vi "Percent to Torque Request.vi"(9 "Enabled":bool, 11 "Throttle %":dbl) -> (2 "MTorqueRequest":sgl)   [LabVIEW 2014]
uses:
  Global Data.vi
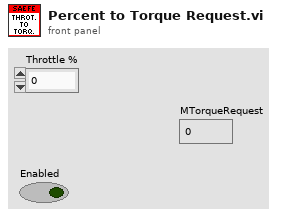
[diagram p1: front panel]
types:
  T1 = typedef "DashDriverInputs.ctl" = cluster{"ButtonsBitArray":u8, "NRedRotary":u8, "NYellowRotary":u8, "NBlackRotary":u8}
  T2 = typedef "MC Position.ctl" = cluster{"aMotor":dbl, "nMotor":dbl, "fMCOutput":dbl, "aDeltaResolverFilt":dbl}
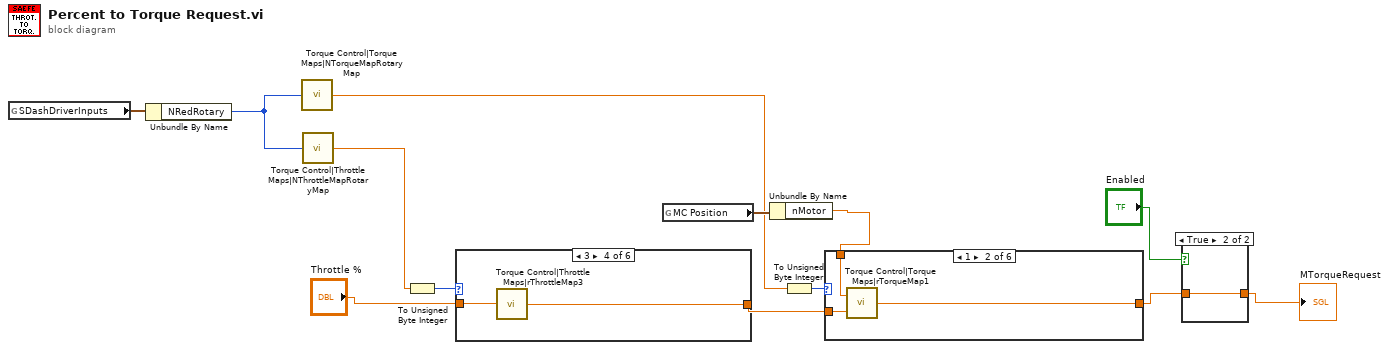
[diagram p0: block diagram]
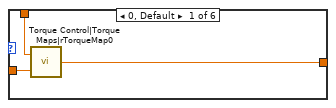
[diagram p2: hidden frame]
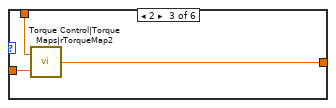
[diagram p3: hidden frame]
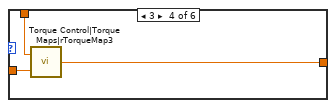
[diagram p4: hidden frame]
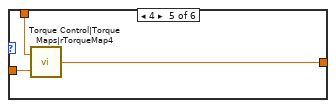
[diagram p5: hidden frame]
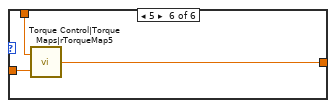
[diagram p6: hidden frame]
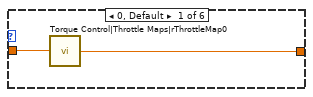
[diagram p7: hidden frame]
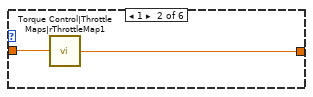
[diagram p8: hidden frame]
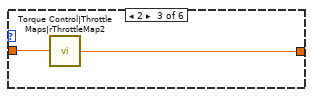
[diagram p9: hidden frame]
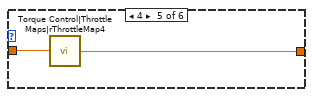
[diagram p10: hidden frame]
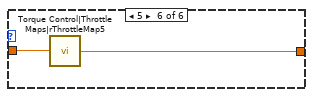
[diagram p11: hidden frame]
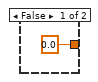
[diagram p12: hidden frame]
diagram:
  n1 = global read "Global Data.vi" "SDashDriverInputs"() -> (w10:T1)
  n2 = Unbundle By Name(w10) -> ("NRedRotary"=w2:u8)
  n3 = call "Torque Control|Torque Maps|NTorqueMapRotaryMap"("X Index"=w2) -> ("Y"=w6:sgl)
  n4 = call "Torque Control|Throttle Maps|NThrottleMapRotaryMap"("X Index"=w2) -> ("Y"=w8:sgl)
  n5 = To Unsigned Byte Integer(number=w8) -> (unsigned 8bit integer=w9:u8)
  n6 = case shown="3" w9 {
    tunnel: "Throttle %" -> [w15 w17 w19 w21 w23 w25]
    tunnel: [w14 w16 w18 w20 w22 w24] -> w11
    frame 0, Default {
      n7 = call "Torque Control|Throttle Maps|rThrottleMap0"("X Index"=w15) -> ("Y"=w14:sgl)
    }
    frame 1 {
      n8 = call "Torque Control|Throttle Maps|rThrottleMap1"("X Index"=w17) -> ("Y"=w16:sgl)
    }
    frame 2 {
      n9 = call "Torque Control|Throttle Maps|rThrottleMap2"("X Index"=w19) -> ("Y"=w18:sgl)
    }
    frame 3 {
      n10 = call "Torque Control|Throttle Maps|rThrottleMap3"("X Index"=w21) -> ("Y"=w20:sgl)
    }
    frame 4 {
      n11 = call "Torque Control|Throttle Maps|rThrottleMap4"("X Index"=w23) -> ("Y"=w22:sgl)
    }
    frame 5 {
      n12 = call "Torque Control|Throttle Maps|rThrottleMap5"("X Index"=w25) -> ("Y"=w24:sgl)
    }
  }
  n13 = global read "Global Data.vi" "MC Position"() -> (w12:T2)
  n14 = Unbundle By Name(w12) -> ("nMotor"=w1:dbl)
  n15 = To Unsigned Byte Integer(number=w6) -> (unsigned 8bit integer=w7:u8)
  n16 = case shown="1" w7 {
    tunnel: w1 -> [w28 w31 w34 w37 w40 w43]
    tunnel: w11 -> [w27 w30 w33 w36 w39 w42]
    tunnel: [w26 w29 w32 w35 w38 w41] -> w4
    frame 0, Default {
      n17 = call "Torque Control|Torque Maps|rTorqueMap0"("Y Index"=w27, "X Index"=w28) -> ("Z"=w26:sgl)
    }
    frame 1 {
      n18 = call "Torque Control|Torque Maps|rTorqueMap1"("Y Index"=w30, "X Index"=w31) -> ("Z"=w29:sgl)
    }
    frame 2 {
      n19 = call "Torque Control|Torque Maps|rTorqueMap2"("Y Index"=w33, "X Index"=w34) -> ("Z"=w32:sgl)
    }
    frame 3 {
      n20 = call "Torque Control|Torque Maps|rTorqueMap3"("Y Index"=w36, "X Index"=w37) -> ("Z"=w35:sgl)
    }
    frame 4 {
      n21 = call "Torque Control|Torque Maps|rTorqueMap4"("Y Index"=w39, "X Index"=w40) -> ("Z"=w38:sgl)
    }
    frame 5 {
      n22 = call "Torque Control|Torque Maps|rTorqueMap5"("Y Index"=w42, "X Index"=w43) -> ("Z"=w41:sgl)
    }
  }
  n23 = case shown="True" "Enabled" {
    tunnel: w4 -> [_ w45]
    tunnel: [0.0 w45] -> w3
    frame False {
    }
    frame True {
    }
  }
  "MTorqueRequest" <- w3
